vi "Set Shooter RPM.vi"(8 "Open Loop":bool, 9 "Increment":bool, 10 "Decrement":bool, 11 "Shooter Enabled":bool) -> ()   [LabVIEW 2012]
uses:
  System Set Points and States.vi
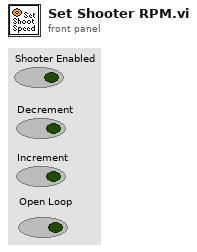
[diagram p1: front panel]
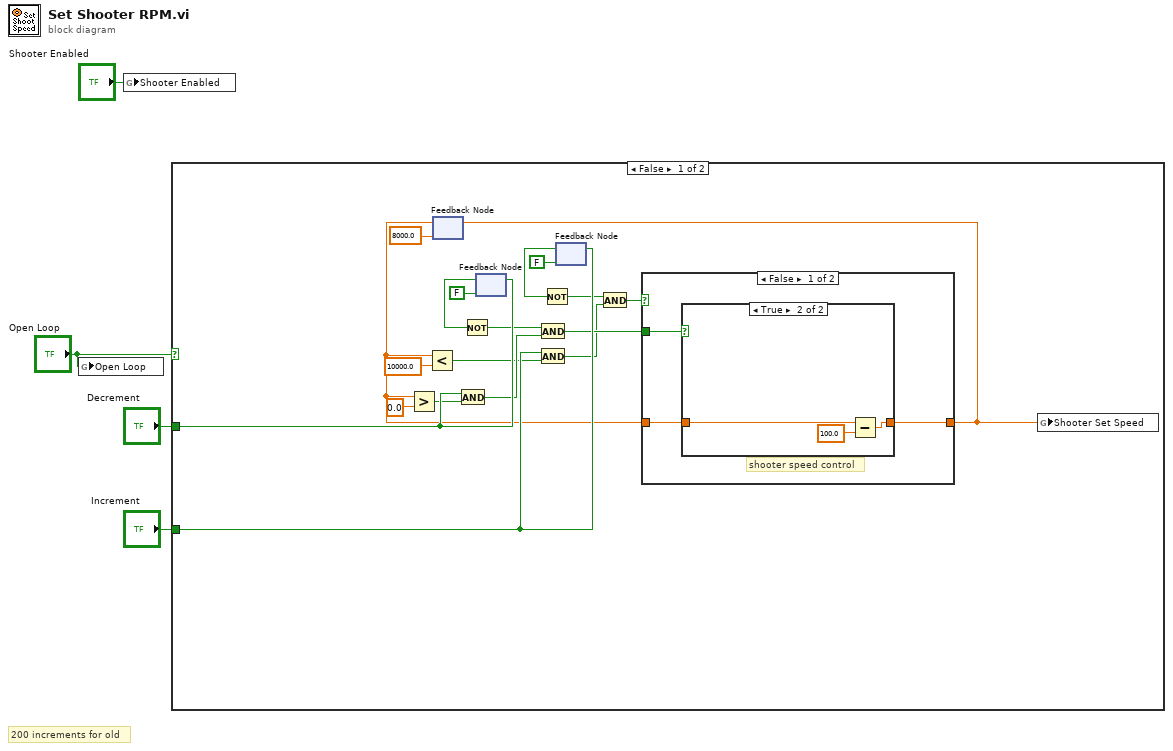
[diagram p0: block diagram]
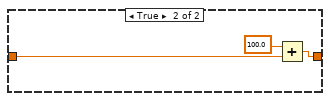
[diagram p3: hidden frame]
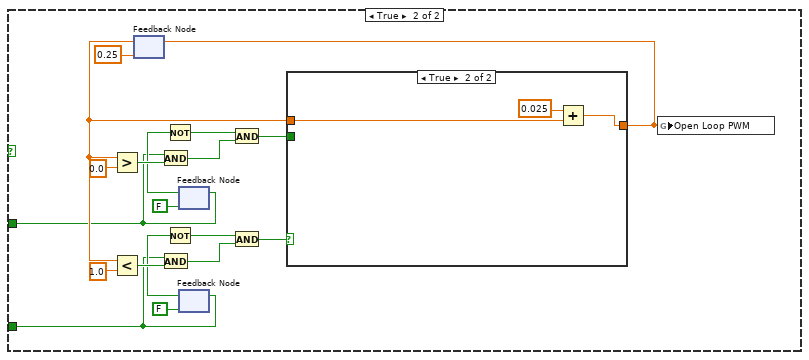
[diagram p4: hidden frame]
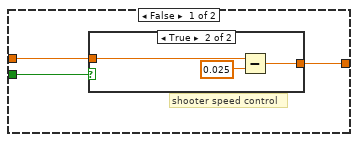
[diagram p5: hidden frame]
diagram:
  # "200 increments for old"
  n1 = global write "System Set Points and States.vi" "Open Loop"("Open Loop") -> ()
  n2 = global write "System Set Points and States.vi" "Shooter Enabled"("Shooter Enabled") -> ()
  n3 = case shown="False" "Open Loop" {
    tunnel: "Decrement" -> [w23 w36]
    tunnel: "Increment" -> [w22 w35]
    frame False {
      n4 = feedback #1(8000.0) -> (w7:dbl)
      n5 = Greater?(x=w7, y=0.0) -> (0:w5:bool)
      n6 = Less?(x=w7, y=10000.0) -> (x < y?=w8:bool)
      n7 = And(x=w23, y=w5) -> (x .and. y?=w14:bool)
      n8 = feedback #2(FALSE) -> (w18:bool)
      n9 = Not(x=w18) -> (.not. x?=w19:bool)
      n10 = feedback-in #2(w23) -> ()
      n11 = And(x=w19, y=w14) -> (x .and. y?=w15:bool)
      n12 = And(x=w22, y=w8) -> (x .and. y?=w11:bool)
      n13 = feedback #3(FALSE) -> (w16:bool)
      n14 = Not(x=w16) -> (.not. x?=w17:bool)
      n15 = feedback-in #3(w22) -> ()
      n16 = And(x=w17, y=w11) -> (x .and. y?=w12:bool)
      n17 = case shown="False" w12 {
        tunnel: w15 -> [w26 _]
        tunnel: w7 -> [w25 w33]
        tunnel: [w24 w31] -> w21
        frame False {
          # "shooter speed control"
          n18 = case shown="True" w26 {
            tunnel: w25 -> [w27 w30]
            tunnel: [w27 w28] -> w24
            frame False {
            }
            frame True {
              n19 = Subtract(x=w30, y=100.0) -> (x-y=w28:dbl)
            }
          }
        }
        frame True {
          n20 = Add(x=100.0, y=w33) -> (x+y=w31:dbl)
        }
      }
      n21 = feedback-in #1(w21) -> ()
      n22 = global write "System Set Points and States.vi" "Shooter Set Speed"(w21) -> ()
    }
    frame True {
      n23 = feedback #4(0.25) -> (w39:dbl)
      n24 = Greater?(x=w39, y=0.0) -> (0:w52:bool)
      n25 = Less?(x=w39, y=1.0) -> (x < y?=w50:bool)
      n26 = And(x=w36, y=w52) -> (x .and. y?=w45:bool)
      n27 = And(x=w35, y=w50) -> (x .and. y?=w47:bool)
      n28 = feedback #5(FALSE) -> (w42:bool)
      n29 = Not(x=w42) -> (.not. x?=w41:bool)
      n30 = feedback-in #5(w36) -> ()
      n31 = feedback #6(FALSE) -> (w44:bool)
      n32 = Not(x=w44) -> (.not. x?=w43:bool)
      n33 = feedback-in #6(w35) -> ()
      n34 = And(x=w41, y=w45) -> (x .and. y?=w38:bool)
      n35 = And(x=w43, y=w47) -> (x .and. y?=w37:bool)
      n36 = case shown="True" w37 {
        tunnel: w38 -> [w55 _]
        tunnel: w39 -> [w54 w62]
        tunnel: [w53 w60] -> w34
        frame False {
          # "shooter speed control"
          n37 = case shown="True" w55 {
            tunnel: w54 -> [w56 w59]
            tunnel: [w56 w57] -> w53
            frame False {
            }
            frame True {
              n38 = Subtract(x=w59, y=0.025) -> (x-y=w57:dbl)
            }
          }
        }
        frame True {
          n39 = Add(x=0.025, y=w62) -> (x+y=w60:dbl)
        }
      }
      n40 = feedback-in #4(w34) -> ()
      n41 = global write "System Set Points and States.vi" "Open Loop PWM"(w34) -> ()
    }
  }
